vi "Automatic Teller Machine (ATM).vi"() -> ()   [LabVIEW 2020]
uses:
  ATM Controller/ATM Controller.lvclass
panel:
  in  "Enter":bool
  in  "User Input":string
  in  "Right Buttons":T1
  out "Right Menu":T2
  in  "Left Buttons":T1
  out "Left Menu":T2
  in  "Card Simulator":bool
  out "ATM Messages":string
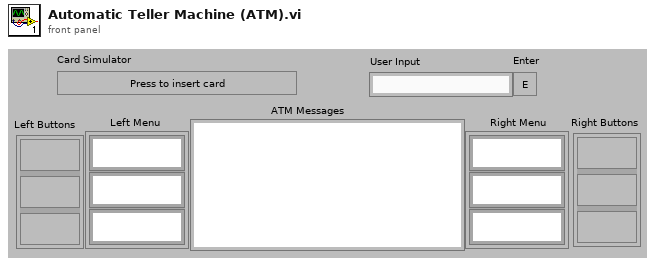
[diagram p1: front panel]
types:
  T1 = cluster{"Func Button":bool, "Func Button 2":bool, "Func Button 3":bool}
  T2 = cluster{"RFS String":string, "RFS String 2":string, "RFS String 3":string}
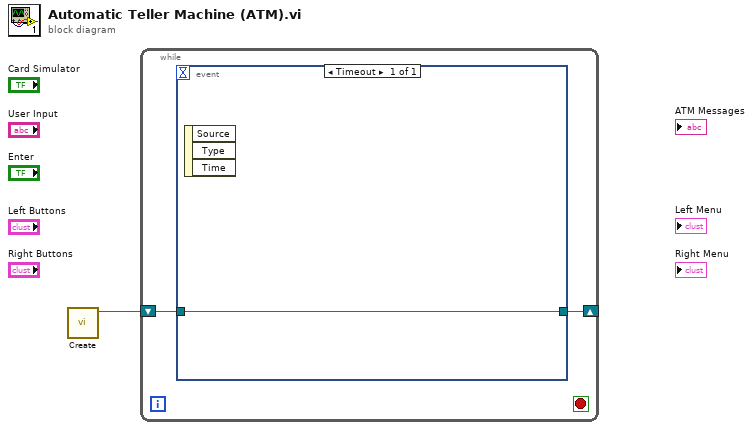
[diagram p0: block diagram]
diagram:
  n1 = call "Create.vi"() -> ("ATM Controller out"=w1:refnum<class "ATM Controller.lvclass">)  [unwired: 10 in, 1 out]
  n2 = while {
    shift-right: [w2] -> _
    shift-left: w1 -> [w3]
    stop <- _ stop-if-true
    n3 = event shown="[0] Timeout" {
      selector: _ -> [_]
      dyn-events: _ -> [_]
      timeout: _ -> [_]
      tunnel: w3 -> [w4]
      tunnel: [w4] -> w2
      event Timeout {
        n4 = event-data() -> ()  [unwired: 1 in, 3 out]
      }
    }
  }
